vi "Robot Systems.vi"(11 "CTR to CMNDS":T1) -> ()   [LabVIEW 2014]
uses:
  JoyStick/Commands.ctl
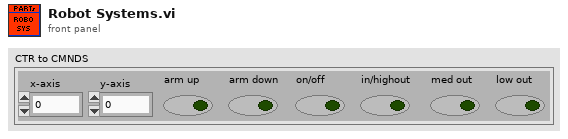
[diagram p1: front panel]
types:
  T1 = typedef "Commands.ctl" = cluster{"x-axis":dbl, "y-axis":dbl, "arm up":bool, "arm down":bool, "on/off":bool, "in/highout":bool, "med out":bool, "low out":bool}
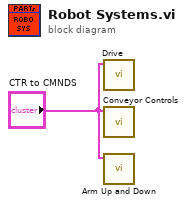
[diagram p0: block diagram]
diagram:
  n1 = call "Drive.vi"("CTR to CMNDS"="CTR to CMNDS") -> ()  [unwired: 11 in]
  n2 = call "Conveyor Controls.vi"("CTR to CMNDS"="CTR to CMNDS") -> ()  [unwired: 11 in]
  n3 = call "Arm Up and Down.vi"("CTR to CMNDS"="CTR to CMNDS") -> ()  [unwired: 11 in]
